vi "HFRR ADV v01.vi"() -> ()   [LabVIEW 2025] (continued)
                  n3919 = Not(x=w4984) -> (.not. x?=w4982:bool)
                  n3920 = Or(x=w4982, y=w4981) -> (x .or. y?=w4983:bool)
                }
              }
            }
          }
          frame #2 {
            w5020 = TRUE ("PAUSE")
            n3921 = call "ELAPSED TIMER VI - demo.vi"("RESET"=w5020, "PAUSE"=w5020) -> ()  [unwired: 7 in, 3 out]
          }
        }
        n3922 = property on="DEMO" class="Bool (strict)"() -> ("Value"=w4852:bool)  [unwired: 2 in, 2 out]
        n3923 = Not(x=w4852) -> (.not. x?=w4851:bool)
        n3924 = Select(t=DEMO_Main_Enum."DEMO STOP", s=w4851, f=w4849) -> (s? t:f=w4848:T18)
      }
      frame "IMAGING" {
        n3925 = flat-sequence {
          tunnel: [w5032] -> w5027
          tunnel: [w5031] -> w5022
          tunnel: w5027 -> [w5042]
          tunnel: [w5042] -> w5026
          tunnel: [w5039] -> w5023
          tunnel: w5022 -> [w5039]
          tunnel: w5026 -> [w5048]
          tunnel: [w5045] -> w5028
          tunnel: [w5044] -> w5024
          tunnel: w5023 -> [w5044]
          tunnel: [w5051] -> w5029
          tunnel: w5028 -> [w5055]
          tunnel: [w5049] -> w5025
          tunnel: w5024 -> [w5050]
          tunnel: [w5068] -> w5030
          tunnel: w5029 -> [w5065]
          tunnel: [w5063] -> _
          tunnel: w5025 -> [w5062]
          frame #0 {
            n3926 = call <vilib>:"Create.vi"("WebView2 Control"="LIVE FEED DISPLAY") -> ("error out"=w5035:errorcluster, "WebView2 Control out"=w5037:refnum<class "WebView2 Control.lvclass">)  [unwired: 9 in]
            n3927 = call <vilib>:"Init Core.vi"("error in (no error)"=w5035, "WebView2 Control in"=w5037) -> ("error out"=w5036:errorcluster, "WebView2 Control out"=w5038:refnum<class "WebView2 Control.lvclass">)  [unwired: 8 in]
            n3928 = call <vilib>:"Write URL.vi"("error in (no error)"=w5036, "uri"="C:\\LAB-IQ\\lib\\VIDEO.html" ("URL"), "WebView2 Control in"=w5038) -> ("error out"=w5032:errorcluster, "WebView2 Control out"=w5031:refnum<class "WebView2 Control.lvclass">)  [unwired: 7 in]
            "error out 4" <- w5032
          }
          frame #1 {
            n3929 = property on="Main Tab" class="TabCtl (strict)"("Value"=T4."Adv Scar" ("Main Tab")) -> ()  [unwired: 2 in, 2 out]
            n3930 = property on="Main Dashboard Buttons" class="RadioBtnsControl (strict)"("Value"=T1."Imaging" ("Main Dashboard Buttons")) -> ()  [unwired: 2 in, 2 out]
          }
          frame #2 {
            n3931 = call <vilib>:"Clear Errors.vi"("error in (no error)"=w5048) -> ("error out"=w5047:errorcluster)  [unwired: 5 in, 1 out]
            n3932 = property on="Magnification len live scar" class="CmbBox"("Value"="10x" ("Magnification len live scar")) -> ()  [unwired: 2 in, 2 out]
            n3933 = property on="FILE 3" class="CmbBox"(error in=w5047, "Value"="DEMO TEST" ("FILE 3")) -> (error out=w5045:errorcluster)  [unwired: 1 in, 1 out]
          }
          frame #3 {
            n3934 = property on="DEMO" class="Bool (strict)"() -> ("Value"=w5053:bool)  [unwired: 2 in, 2 out]
            n3935 = Not(x=w5053) -> (.not. x?=w5052:bool)
            n3936 = case shown="False" w5052 {
              tunnel: w5055 -> [w5058 w5059]
              tunnel: [w5057 w5059] -> w5054
              frame False {
                n3937 = call "Stall Data Flow.vim"("value in"=w5058, "milliseconds to wait"="LIVE FEED DELAY") -> ("value out"=w5057:errorcluster)  [unwired: 1 out]
              }
              frame True {
              }
            }
            n3938 = call <vilib>:"Stop.vi"("error in (no error)"=w5054, "WebView2 Control in"=w5050) -> ("error out"=w5051:errorcluster, "WebView2 Control out"=w5049:refnum<class "WebView2 Control.lvclass">)  [unwired: 8 in]
          }
          frame #4 {
            n3939 = call "Stall Data Flow.vim"("value in"=w5065, "milliseconds to wait"=u32 2000) -> ("value out"=w5061:errorcluster)  [unwired: 1 out]
            n3940 = property on="Main Tab" class="TabCtl (strict)"("Value"=T4."Adv Scar Report" ("Main Tab")) -> ()  [unwired: 2 in, 2 out]
            n3941 = call <vilib>:"Dispose.vi"("error in (no error)"=w5061, "WebView2 Control in"=w5062) -> ("error out"=w5064:errorcluster)  [unwired: 9 in]
            n3942 = property on="Main Dashboard Buttons" class="RadioBtnsControl (strict)"("Value"=T1."Report" ("Main Dashboard Buttons")) -> ()  [unwired: 2 in, 2 out]
            n3943 = property on="DEMO" class="Bool (strict)"() -> ("Value"=w5072:bool)  [unwired: 2 in, 2 out]
            n3944 = Not(x=w5072) -> (.not. x?=w5071:bool)
            n3945 = Select(t=DEMO_Main_Enum."DEMO STOP", s=w5071, f=DEMO_Main_Enum."REPORT") -> (s? t:f=w5068:T18)
            n3946 = call <vilib>:"Clear Errors.vi"("error in (no error)"=w5064) -> ("error out"=w5063:errorcluster)  [unwired: 5 in, 1 out]
          }
        }
      }
      frame "REPORT" {
        n3947 = flat-sequence {
          tunnel: [w5082] -> w5080
          tunnel: [w5081] -> w5077
          tunnel: w5080 -> [w5091]
          tunnel: [w5090] -> w5079
          tunnel: w5077 -> [w5089]
          tunnel: [w5089] -> w5076
          tunnel: w5079 -> [w5100]
          tunnel: [w5094] -> w5078
          tunnel: w5076 -> [w5099]
          tunnel: [w5096] -> w5075
          tunnel: w5078 -> [w5114]
          tunnel: w5075 -> [w5109]
          tunnel: [w5108] -> w5073
          tunnel: [DEMO_Main_Enum."DEMO STOP"] -> w5074
          tunnel: [w5116] -> _
          tunnel: w5073 -> [w5116]
          frame #0 {
            n3948 = call <vilib>:"Create.vi"("WebView2 Control"="LIVE FEED DISPLAY 2") -> ("error out"=w5085:errorcluster, "WebView2 Control out"=w5087:refnum<class "WebView2 Control.lvclass">)  [unwired: 9 in]
            n3949 = call <vilib>:"Init Core.vi"("error in (no error)"=w5085, "WebView2 Control in"=w5087) -> ("error out"=w5086:errorcluster, "WebView2 Control out"=w5088:refnum<class "WebView2 Control.lvclass">)  [unwired: 8 in]
            n3950 = call <vilib>:"Write URL.vi"("error in (no error)"=w5086, "uri"="C:\\LAB-IQ\\lib\\POST ANALYSIS.html" ("URL"), "WebView2 Control in"=w5088) -> ("error out"=w5082:errorcluster, "WebView2 Control out"=w5081:refnum<class "WebView2 Control.lvclass">)  [unwired: 7 in]
          }
          frame #1 {
            n3951 = local write "Magnification :"("10x" ("Magnification :")) -> ()
            n3952 = property on="Test File List :" class="CmbBox"(error in=w5091, "Value"="DEMO TEST" ("FILE 3")) -> (error out=w5090:errorcluster)  [unwired: 1 in, 1 out]
          }
          frame #2 {
            n3953 = property on="DEMO" class="Bool (strict)"() -> ("Value"=w5098:bool)  [unwired: 2 in, 2 out]
            n3954 = Not(x=w5098) -> (.not. x?=w5097:bool)
            n3955 = case shown="False" w5097 {
              tunnel: w5100 -> [w5103 w5104]
              tunnel: [w5102 w5104] -> w5095
              frame False {
                n3956 = call "Stall Data Flow.vim"("value in"=w5103, "milliseconds to wait"=u32 11000) -> ("value out"=w5102:errorcluster)  [unwired: 1 out]
              }
              frame True {
              }
            }
            n3957 = call <vilib>:"Stop.vi"("error in (no error)"=w5095, "WebView2 Control in"=w5099) -> ("error out"=w5094:errorcluster, "WebView2 Control out"=w5096:refnum<class "WebView2 Control.lvclass">)  [unwired: 8 in]
          }
          frame #3 {
            n3958 = call "Stall Data Flow.vim"("value in"=w5114, "milliseconds to wait"=u32 2000) -> ("value out"=w5106:errorcluster)  [unwired: 1 out]
            n3959 = call <vilib>:"Dispose.vi"("error in (no error)"=w5106, "WebView2 Control in"=w5109) -> ("error out"=w5110:errorcluster)  [unwired: 9 in]
            n3960 = local write "Major Axis"(345.9 ("Major Axis")) -> ()
            n3961 = local write "Minor Axis"(422.3 ("Minor Axis")) -> ()
            n3962 = local write "Average"(384.1 ("Average")) -> ()
            n3963 = call "Stall Data Flow.vim"("value in"=w5110, "milliseconds to wait"=u32 1500) -> ("value out"=w5108:errorcluster)  [unwired: 1 out]
          }
          frame #4 {
          }
        }
      }
      frame "DEMO STOP" {
        w5117 = 0.0 ("Average")
        w5118 = "" ("FILE 3")
        w5123 = "" ("USERNAME")
        n3964 = property on="USERNAME" class="Str"("Value"=w5123) -> ()  [unwired: 2 in, 2 out]
        n3965 = property on="USER ID" class="Str"("Value"=w5123) -> ()  [unwired: 2 in, 2 out]
        n3966 = property on="FILE" class="Str"("Value"=w5123) -> ()  [unwired: 2 in, 2 out]
        n3967 = property on="Batch Ref Num :" class="Str"("Value"=w5123) -> ()  [unwired: 2 in, 2 out]
        n3968 = property on="tested by" class="Str"("Value"=w5123) -> ()  [unwired: 2 in, 2 out]
        n3969 = property on="Fuel Discription :" class="Str"("Value"=w5123) -> ()  [unwired: 2 in, 2 out]
        n3970 = property on="Remarks :" class="Str"("Value"=w5123) -> ()  [unwired: 2 in, 2 out]
        n3971 = property on="OPERATOR ID" class="Str"("Value"=w5123) -> ()  [unwired: 2 in, 2 out]
        n3972 = property on="Auto Start Test" class="Bool (strict)"("Value"=FALSE ("Auto Start Test")) -> ()  [unwired: 2 in, 2 out]
        n3973 = property on="RUN" class="Bool (strict)"("Visible"=TRUE) -> ()  [unwired: 2 in, 2 out]
        n3974 = property on="Main Dashboard Buttons" class="RadioBtnsControl (strict)"("Value"=T1."Home" ("Main Dashboard Buttons")) -> ()  [unwired: 2 in, 2 out]
        n3975 = property on="Main Tab" class="TabCtl (strict)"("Value"=T4."HOME" ("Main Tab")) -> ()  [unwired: 2 in, 2 out]
        n3976 = property on="main tab sub" class="TabCtl (strict)"("Value"=enum32{"Page 1", "Page 2"}."Page 1" ("main tab sub")) -> ()  [unwired: 2 in, 2 out]
        n3977 = local write "Magnification :"("5x" ("Magnification :")) -> ()
        n3978 = local write "Major Axis"(w5117) -> ()
        n3979 = local write "Minor Axis"(w5117) -> ()
        n3980 = local write "Average"(w5117) -> ()
        n3981 = property on="FILE 3" class="CmbBox"("Value"=w5118) -> ()  [unwired: 2 in, 2 out]
        n3982 = property on="Test File List :" class="CmbBox"("Value"=w5118) -> ()  [unwired: 2 in, 2 out]
        n3983 = property on="Magnification len live scar" class="CmbBox"("Value"=w5118) -> ()  [unwired: 2 in, 2 out]
      }
    }
    n3984 = local read "Quit"() -> (w4788:bool)
  }
  n3985 = while {
    stop <- w5128 stop-if-true
    n3986 = call <vilib>:"High Resolution Polling Wait.vi"("seconds to wait"=0.05) -> ()  [unwired: 10 in, 1 out]
    n3987 = disable-structure shown="Enabled" {
      frame Disabled {
        n3988 = local read "Read HUMIDITY"() -> (w5129:string)
        n3989 = Spreadsheet String To Array(delimiter (Tab)=",", format string="", spreadsheet string=w5129, array type (2D Dbl)=string[] []) -> (array=w5148:string[])
        n3990 = for {
          tunnel: w5148 -> [w5157] mode=indexing
          tunnel: string[] ["STATE;", "SET;", "RH;", "T;", "AMB_RH;", "AMB_T;", "PUMP;", "FAN_IN;", "FAN_OUT;", "DEHUM;", "CURRENT;", "STALL;"] -> [w5156] mode=indexing
          tunnel: [w5155] -> w5147 mode=indexing
          n3991 = Match Pattern(string=w5157, regular expression=w5156) -> (after substring=w5155:string)  [unwired: 1 in, 3 out]
        }
        n3992 = Index Array(array=w5147) -> (element #1=w5146:string, element #2=w5145:string, element #3=w5137:string, element #4=w5136:string, element #5=w5135:string, element #6=w5144:string, element #7=w5143:string, element #8=w5142:string, element #9=w5141:string, element #10=w5140:string, element #11=w5139:string, element #12=w5138:string)  [unwired: 12 in]
        n3993 = Fract/Exp String To Number(string=w5137) -> (number=w5130:dbl)  [unwired: 3 in, 1 out]
        n3994 = Fract/Exp String To Number(string=w5135) -> (number=w5134:dbl)  [unwired: 3 in, 1 out]
        n3995 = local write "Ambient Humidity :"(w5134) -> ()
        n3996 = Equal?(x=w5130, y=0.0) -> (x = y?=w5132:bool)
        n3997 = case shown="True" w5132 {
          tunnel: [w5153 w5154] -> w5131
          tunnel: w5130 -> [w5153 _]
          frame False {
            (unwired) 0.0
            "Humidity temp" <- w5153
          }
          frame True {
            n3998 = local read "Humidity temp"() -> (w5154:dbl)
          }
        }
        "RH Numeric:" <- w5131
      }
      frame Enabled {
        n3999 = local read "Read HUMIDITY"() -> (w5177:string)
        n4000 = Spreadsheet String To Array(delimiter (Tab)=",", format string="", spreadsheet string=w5177, array type (2D Dbl)=dbl[] []) -> (array=w5173:dbl[])
        n4001 = Index Array(array=w5173) -> (element #1=→"STATE :":dbl, element #2=→"SET :":dbl, element #3=w5158:dbl, element #4=→"T :":dbl, element #5=→"AMB_RH :":dbl, element #6=→"AMB_T :":dbl, element #7=→"PUMP :":dbl, element #8=→"FAN_IN :":dbl, element #9=→"FAN_OUT :":dbl, element #10=→"DEHUM :":dbl, element #11=→"CURRENT :":dbl, element #12=→"STALL":dbl)  [unwired: 12 in]
        "RH :" <- w5158
        n4002 = Equal?(x=w5158, y=0.0) -> (x = y?=w5161:bool)
        n4003 = case shown="False" w5161 {
          tunnel: [w5178 w5179] -> w5162
          tunnel: w5158 -> [w5178 _]
          frame False {
            "Humidity temp 2" <- w5178
          }
          frame True {
            n4004 = local read "Humidity temp 2"() -> (w5179:dbl)
          }
        }
        n4005 = local write "RH Numeric:"(w5162) -> ()
      }
    }
    n4006 = local read "Quit"() -> (w5128:bool)
  }
  n4007 = while {
    shift-right: [w5185] -> _
    shift-left: _ -> [w5186]
    shift-right: [w5183] -> _
    shift-left: T21 {"Read Uno"="", "Bytes at Heave Port"=0.0, "UNO COM Port:"="COM9", "UNO COM Port: 2"="COM7", "Residual Due"="", "UNO COM Status 2"=TRUE, "UNO COM Status"=TRUE, "Port 2"=TRUE, "Sway PPR"=6400.0, "Surge PPR"=6400.0, "Heave PPR"=6400.0, "Sway Pitch"=2.0, "Surge Pitch"=3.0, "Heave Pitch"=4.0, "Sway Pulses/mm"=320.0, "Surge Pulses/mm"=1600.0, "Heave Pulses/mm"=1600.0, "inner loop"=0.0, "Read Heave and Surge 2"="", "String 36"="", "Write S"=FALSE, "WriteCC1"=[""], "Heave COM Loop"=0, "LastCom"="", "EXIT"=FALSE, "Error Heave"={"status"=TRUE, "code"=-1073807343, "source"=""}} -> [w5182]
    shift-right: [w5180] -> _
    shift-left: enum16{"init", "MAIN", "Panel Close"}."init" -> [w5181]
    stop <- w5184 stop-if-true
    # "UNO CODE LOGIC"
    n4008 = case shown="\"init\"" w5181 {
      tunnel: w5186 -> [w5200 w5223 w5293 w5295]
      tunnel: [w5195 w5209 w5293 w5295] -> w5185
      tunnel: [_ _ TRUE _] -> w5184
      tunnel: [w5191 w5208 w5291 w5294] -> w5183
      tunnel: w5182 -> [w5197 w5222 w5291 w5294]
      tunnel: [enum16{"init", "MAIN", "Panel Close"}."MAIN" w5217 _ _] -> w5180
      frame "init" {
        n4009 = local read "Com Port 1"() -> (w5187:refnum<visa-resource-name>)
        n4010 = Bundle By Name(cluster=w5197, "UNO COM Port:"=w5187) -> (w5196:T21)
        n4011 = call "Instrument fgv.vi"("Enum"=T32."INIT", "error in (no error) 2"=w5200, "INPUT"=w5196) -> ("error"=w5198:errorcluster, "output"=w5194:T19)  [unwired: 6 in, 1 out]
        n4012 = case shown="Error" w5198 {
          selector: w5198 -> [w5202 _]
          tunnel: [w5202 w5206] -> w5195
          tunnel: w5194 -> [w5201 w5204]
          tunnel: [w5201 w5203] -> w5192
          frame No Error {
          }
          frame Error {
            n4013 = call "Instrument fgv.vi"("Enum"=T32."ERROR INIT", "INPUT"=w5204) -> ("error"=w5207:errorcluster, "output"=w5203:T19)  [unwired: 7 in, 1 out]
            n4014 = call <vilib>:"Clear Errors.vi"("error in (no error)"=w5207) -> ("error out"=w5206:errorcluster)  [unwired: 5 in, 1 out]
          }
        }
        n4015 = local read "LastCom UNO"() -> (w5189:string)
        n4016 = Unbundle By Name(w5192) -> ("Heave COM Status 2"=→"Instrument Status":bool, "Error Heave"=→"Error  2":errorcluster)  [unwired: 1 out]
        n4017 = Bundle By Name(cluster=w5192, "LastCom"=w5189) -> (w5191:T19)
      }
      frame "MAIN" {
        n4018 = Unbundle By Name(w5222) -> ("UNO COM Port: 2"=w5212:refnum<visa-resource-name>)
        n4019 = local read "Com Port 1"() -> (w5213:refnum<visa-resource-name>)
        n4020 = local write "COM Port UNO :"(w5212) -> ()
        n4021 = Equal?(x=w5212, y=w5213) -> (x = y?=w5227:bool)
        n4022 = Bundle By Name(cluster=w5222, "UNO COM Port:"=w5213) -> (w5221:T21)
        n4023 = case shown="True" w5227 {
          tunnel: [w5247 w5264] -> w5211
          tunnel: w5223 -> [w5248 w5270]
          tunnel: w5221 -> [w5246 w5268]
          tunnel: [w5245 w5263] -> w5210
          frame False {
            n4024 = call <vilib>:"Clear Errors.vi"("error in (no error)"=w5248) -> ("error out"=w5244:errorcluster)  [unwired: 5 in, 1 out]
            n4025 = call "Instrument fgv.vi"("Enum"=T32."ERROR INIT", "error in (no error) 2"=w5244, "INPUT"=w5246) -> ("error"=w5250:errorcluster, "output"=w5245:T19)  [unwired: 6 in, 1 out]
            n4026 = call <vilib>:"Clear Errors.vi"("error in (no error)"=w5250) -> ("error out"=w5247:errorcluster)  [unwired: 5 in, 1 out]
          }
          frame True {
            n4027 = call "Instrument fgv.vi"("Enum"=T32."READ", "error in (no error) 2"=w5270, "INPUT"=w5268) -> ("error"=w5269:errorcluster, "output"=w5262:T19)  [unwired: 6 in, 1 out]
            n4028 = Bundle By Name(cluster=w5262, "String 36"="WRITE UNO") -> (w5261:T19)
            n4029 = case shown="True" "Write" {
              selector: "Write" -> [_ w5285]
              tunnel: w5269 -> [w5283 w5290]
              tunnel: [w5283 w5289] -> w5259
              tunnel: w5261 -> [w5282 w5287]
              tunnel: [w5282 w5286] -> w5258
              frame False {
              }
              frame True {
                n4030 = Not(x=w5285) -> (.not. x?=w5284:bool)
                n4031 = local write "Write"(w5284) -> ()
                n4032 = call "Instrument fgv.vi"("Enum"=T32."MANUAL WRITE", "error in (no error) 2"=w5290, "INPUT"=w5287) -> ("error"=w5289:errorcluster, "output"=w5286:T19)  [unwired: 6 in, 1 out]
              }
            }
            n4033 = Array Size(array="Write UNO") -> (size(s)=w5256:i32)
            n4034 = Greater Than 0?(x=w5256) -> (x > 0?=w5255:bool)
            n4035 = call "Instrument fgv.vi"("Enum"=T32."WRITE", "error in (no error) 2"=w5259, "WriteCC1"="Write UNO", "INPUT"=w5258) -> ("error"=w5266:errorcluster, "WriteCC1 2"=w5257:string[], "output"=w5265:T19)  [unwired: 5 in]
            n4036 = case shown="True" w5255 {
              tunnel: w5257 -> [_ w5272]
              frame False {
              }
              frame True {
                n4037 = local write "Write UNO"(w5272) -> ()
              }
            }
            n4038 = case shown="Error" w5266 {
              selector: w5266 -> [w5273 w5276]
              tunnel: w5265 -> [w5274 w5281]
              tunnel: [w5274 w5280] -> w5263
              tunnel: [w5273 w5278] -> w5264
              frame No Error {
              }
              frame Error {
                n4039 = call <vilib>:"Clear Errors.vi"("error in (no error)"=w5276) -> ("error out"=w5275:errorcluster)  [unwired: 5 in, 1 out]
                n4040 = call "Instrument fgv.vi"("Enum"=T32."ERROR INIT", "error in (no error) 2"=w5275, "INPUT"=w5281) -> ("error"=w5279:errorcluster, "output"=w5280:T19)  [unwired: 6 in, 1 out]
                n4041 = call <vilib>:"Clear Errors.vi"("error in (no error)"=w5279) -> ("error out"=w5278:errorcluster)  [unwired: 5 in, 1 out]
              }
            }
            n4042 = Unbundle By Name(w5263) -> ("LastCom"=→"LastCom UNO":string, "Read Heave and Surge"=→"Read UNO":string)
          }
        }
        n4043 = Unbundle By Name(w5210) -> ("Heave COM Status 2"=w5226:bool, "Heave COM Status"=w5216:bool, "Error Heave"=w5214:errorcluster, "Bytes at Heave Port"=→"Bytes at Uno":dbl)
        n4044 = Not(x=w5216) -> (.not. x?=w5224:bool)
        n4045 = Not(x=w5226) -> (.not. x?=w5215:bool)
        n4046 = local write "Instrument Status"(w5224) -> ()
        n4047 = local write "Error  2"(w5214) -> ()
        n4048 = local write "Port 1a"(w5216) -> ()
        n4049 = local read "Quit"() -> (w5218:bool)
        n4050 = local write "COM Status"(w5215) -> ()
        n4051 = Select(t=enum16{"init", "MAIN", "Panel Close"}."Panel Close", s=w5218, f=enum16{"init", "MAIN", "Panel Close"}."MAIN") -> (s? t:f=w5217:enum16{"init", "MAIN", "Panel Close"})
        n4052 = case shown="No Error" w5211 {
          tunnel: w5211 -> [w5231 w5243]
          tunnel: w5210 -> [w5230 w5242]
          tunnel: [w5229 w5243] -> w5209
          tunnel: [w5228 w5242] -> w5208
          frame No Error {
            n4053 = First Call?() -> (First Call?: T/F=w5232:bool)
            n4054 = case shown="True" w5232 {
              tunnel: w5230 -> [w5234 w5241]
              tunnel: [w5234 w5240] -> w5228
              tunnel: [w5233 w5238] -> w5229
              tunnel: w5231 -> [w5233 w5235]
              frame False {
              }
              frame True {
                n4055 = call <vilib>:"Clear Errors.vi"("error in (no error)"=w5235) -> ("error out"=w5236:errorcluster)  [unwired: 5 in, 1 out]
                n4056 = call "Instrument fgv.vi"("Enum"=T32."ERROR INIT", "error in (no error) 2"=w5236, "INPUT"=w5241) -> ("error"=w5239:errorcluster, "output"=w5240:T19)  [unwired: 6 in, 1 out]
                n4057 = call <vilib>:"Clear Errors.vi"("error in (no error)"=w5239) -> ("error out"=w5238:errorcluster)  [unwired: 5 in, 1 out]
              }
            }
          }
          frame Error {
          }
        }
      }
      frame "Panel Close" {
      }
      frame Default {
      }
    }
  }
